vi "Get Source Wfm Refs.vi"(8 "Error in":errorcluster, 11 "Device Ref in":T2 format="%.0x") -> (0 "Error out":errorcluster, 3 "Device Ref out":T2=18446744073709551615 format="%.0x", 5 "Source Wfm Data Refs":T1[](array[typedef]))   [LabVIEW 2015, in "Waveform-Processing-Custom-Device System Explorer.lvlib"]
uses:
  Waveform-Processing-Custom-Device System Explorer.lvlib
  <vilib>/NI Veristand/Custom Device API/Custom Device Item Ref.ctl
  <vilib>/NI Veristand/Custom Device API/Waveform Data Reference.ctl
  Shared/Constants.vi
  <vilib>/NI Veristand/Custom Device API/Get Item Property (Dependent Node Pointer).vi
  <vilib>/NI VeriStand/Custom Device API/Custom Device API.lvlib
  Shared/Waveform-Processing-Custom-Device Shared.lvlib
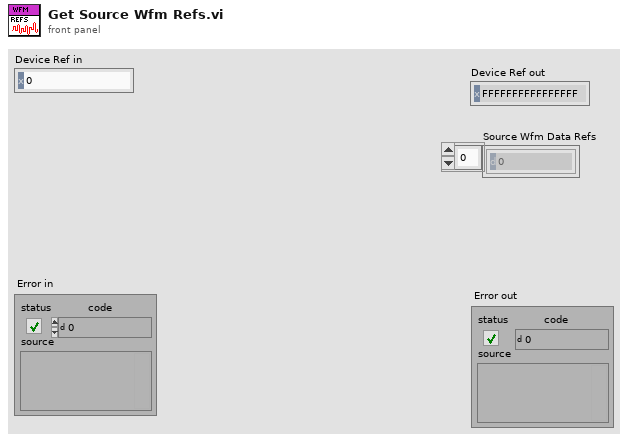
[diagram p1: front panel]
types:
  T1 = typedef "Custom Device API.lvlib/Waveform Data Reference.ctl" = i32
  T2 = typedef "Custom Device API.lvlib/Custom Device Item Ref.ctl" = u64
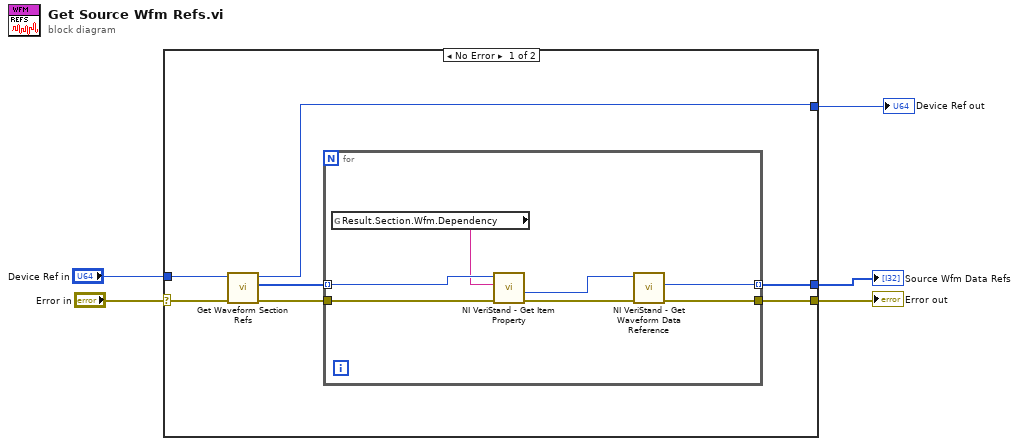
[diagram p0: block diagram]
diagram:
  n1 = case shown="No Error" "Error in" {
    selector: "Error in" -> [w12 w21]
    tunnel: [w7 w21] -> w4
    tunnel: "Device Ref in" -> [w11 w20]
    tunnel: [w8 w20] -> w2
    tunnel: [w6 _] -> w1
    frame No Error {
      n2 = call "Get Waveform Section Refs.vi"("Error in"=w12, "Device Ref in"=w11) -> ("Error out"=w10:errorcluster, "Result Section Refs"=w9:T2[], "Device Ref out"=w8:T2)  [unwired: 7 in]
      n3 = for {
        tunnel: w10 -> [w19]
        tunnel: w9 -> [w18] mode=indexing
        tunnel: [w15] -> w7
        tunnel: [w13] -> w6 mode=indexing
        n4 = global read "Constants.vi" "Result.Section.Wfm.Dependency"() -> (w17:string)
        n5 = call-poly <vilib>:"NI VeriStand - Get Item Property.vi"("error in (no error)"=w19, "Property Name"=w17, "Item Ref in"=w18) -> ("error out"=w16:errorcluster, "Dependent Node Ref"=w14:T2)  [unwired: 5 in, 2 out]
        n6 = call <vilib>:"NI VeriStand - Get Waveform Data Reference.vi"("error in (no error)"=w16, "Waveform Ref in"=w14) -> ("error out"=w15:errorcluster, "Waveform Data Reference"=w13:T1)  [unwired: 7 in, 1 out]
      }
    }
    frame Error {
    }
  }
  "Error out" <- w4
  "Device Ref out" <- w2
  "Source Wfm Data Refs" <- w1
